vi "Autonomous Independent 3-17-15.vi"() -> ()   [LabVIEW 2014]
doc: "This VI is called when autonomous begins, and will automatically be terminated when autonomous ends. You can carry out timed or sensor driven robot movement independently without needing to return to the caller."
uses:
  Dashboard/Autonomous Type.ctl
  <vilib>/Rock Robotics/WPI/Joystick/WPI_JoystickGetSetRefNum.vi
  <vilib>/Rock Robotics/Network Tables/SD Write Numeric Array.vi
  <vilib>/Rock Robotics/WPI/RobotDrive/WPI_RobotDriveGetSetRefNum.vi
  <vilib>/Rock Robotics/Network Tables/SD Read Number.vi
  <vilib>/Rock Robotics/Network Tables/SD Write String.vi
  <vilib>/Rock Robotics/WPI/RobotDrive/WPI_RobotDriveMecanumDrive_Cartesian.vi
panel:
  in  "3 totes strafe":T1(array[cluster])=[{"X Joystick Value"=-0.3, "Y Joystick Value"=-1.0, "Z Joystick Value"=0.0, "Delay (sec)"=1.0, "Movement Name"="", "Mode"=enum."Move Robot"}, {"X Joystick Value"=0.3, "Y Joystick Value"=0.0, "Z Joystick Value"=0.0, "Delay (sec)"=0.25, "Movement Name"="", "Mode"=enum."Lift Tote"}, {"X Joystick Value"=0.0, "Y Joystick Value"=-0.5, "Z Joystick Value"=0.0, "Delay (sec)"=1.0, "Movement Name"="", "Mode"=enum."Move Robot"}, {"X Joystick Value"=0.0, "Y Joystick Value"=0.0, "Z Joystick Value"=0.0, "Delay (sec)"=4.0, "Movement Name"="", "Mode"=enum."Lift Tote"}, {"X Joystick Value"=0.0, "Y Joystick Value"=0.3, "Z Joystick Value"=0.0, "Delay (sec)"=1.0, "Movement Name"="", "Mode"=enum."Move Robot"}, {"X Joystick Value"=0.5353535353535355, "Y Joystick Value"=0.0, "Z Joystick Value"=0.0, "Delay (sec)"=1.0, "Movement Name"="", "Mode"=enum."Move Robot"}, {"X Joystick Value"=0.0, "Y Joystick Value"=-0.3, "Z Joystick Value"=0.0, "Delay (sec)"=0.251, "Movement Name"="", "Mode"=enum."Move Robot"}, {"X Joystick Value"=-0.3, "Y Joystick Value"=0.0, "Z Joystick Value"=0.0, "Delay (sec)"=1.0, "Movement Name"="", "Mode"=enum."Move Robot"}, {"X Joystick Value"=0.3, "Y Joystick Value"=0.0, "Z Joystick Value"=0.0, "Delay (sec)"=0.25, "Movement Name"="", "Mode"=enum."Move Robot"}, {"X Joystick Value"=0.0, "Y Joystick Value"=-0.5, "Z Joystick Value"=0.0, "Delay (sec)"=0.0, "Movement Name"="", "Mode"=enum."Move Robot"}, {"X Joystick Value"=0.0, "Y Joystick Value"=0.0, "Z Joystick Value"=0.0, "Delay (sec)"=3.5, "Movement Name"="", "Mode"=enum."Lift Tote"}, {"X Joystick Value"=0.0, "Y Joystick Value"=0.3, "Z Joystick Value"=0.0, "Delay (sec)"=3.5, "Movement Name"="", "Mode"=enum."Move Robot"}, {"X Joystick Value"=0.3, "Y Joystick Value"=0.0, "Z Joystick Value"=0.0, "Delay (sec)"=0.0, "Movement Name"="", "Mode"=enum."Move Robot"}, {"X Joystick Value"=0.0, "Y Joystick Value"=-0.5, "Z Joystick Value"=0.0, "Delay (sec)"=0.0, "Movement Name"="", "Mode"=enum."Move Robot"}, {"X Joystick Value"=-0.3, "Y Joystick Value"=0.0, "Z Joystick Value"=0.0, "Delay (sec)"=0.0, "Movement Name"="", "Mode"=enum."Move Robot"}, {"X Joystick Value"=0.3, "Y Joystick Value"=0.0, "Z Joystick Value"=0.0, "Delay (sec)"=0.0, "Movement Name"="", "Mode"=enum."Move Robot"}, {"X Joystick Value"=0.0, "Y Joystick Value"=-0.5, "Z Joystick Value"=0.0, "Delay (sec)"=0.0, "Movement Name"="", "Mode"=enum."Do Nothing"}, {"X Joystick Value"=0.0, "Y Joystick Value"=0.0, "Z Joystick Value"=0.0, "Delay (sec)"=0.0, "Movement Name"="", "Mode"=enum."Lift Tote"}, {"X Joystick Value"=0.0, "Y Joystick Value"=0.5, "Z Joystick Value"=0.0, "Delay (sec)"=0.0, "Movement Name"="", "Mode"=enum."Move Robot"}] {"Z Joystick Value" scale=-1.0..1.0; "Y Joystick Value" scale=1.0..-1.0; "X Joystick Value" scale=-1.0..1.0}
  in  "2 totes + turn":T1(array[cluster])=[{"X Joystick Value"=-0.3, "Y Joystick Value"=0.0, "Z Joystick Value"=0.0, "Delay (sec)"=1.0, "Movement Name"="", "Mode"=enum."Move Robot"}, {"X Joystick Value"=0.3, "Y Joystick Value"=0.0, "Z Joystick Value"=0.0, "Delay (sec)"=0.25, "Movement Name"="", "Mode"=enum."Move Robot"}, {"X Joystick Value"=0.0, "Y Joystick Value"=-0.5, "Z Joystick Value"=0.0, "Delay (sec)"=1.0, "Movement Name"="", "Mode"=enum."Move Robot"}, {"X Joystick Value"=0.0, "Y Joystick Value"=0.0, "Z Joystick Value"=0.0, "Delay (sec)"=4.0, "Movement Name"="", "Mode"=enum."Lift Tote"}, {"X Joystick Value"=0.0, "Y Joystick Value"=0.3, "Z Joystick Value"=0.0, "Delay (sec)"=0.30000000000000004, "Movement Name"="", "Mode"=enum."Move Robot"}, {"X Joystick Value"=0.0, "Y Joystick Value"=0.0, "Z Joystick Value"=0.677190686694989, "Delay (sec)"=2.0, "Movement Name"="", "Mode"=enum."Move Robot"}, {"X Joystick Value"=0.0, "Y Joystick Value"=-0.5, "Z Joystick Value"=0.0, "Delay (sec)"=2.0, "Movement Name"="", "Mode"=enum."Move Robot"}, {"X Joystick Value"=0.0, "Y Joystick Value"=0.0, "Z Joystick Value"=-0.6724763557187154, "Delay (sec)"=1.0, "Movement Name"="", "Mode"=enum."Move Robot"}, {"X Joystick Value"=0.0, "Y Joystick Value"=-0.5, "Z Joystick Value"=0.0, "Delay (sec)"=0.25, "Movement Name"="", "Mode"=enum."Move Robot"}, {"X Joystick Value"=-0.3, "Y Joystick Value"=0.0, "Z Joystick Value"=0.0, "Delay (sec)"=1.0, "Movement Name"="", "Mode"=enum."Move Robot"}, {"X Joystick Value"=0.3, "Y Joystick Value"=0.0, "Z Joystick Value"=0.0, "Delay (sec)"=0.0, "Movement Name"="", "Mode"=enum."Move Robot"}, {"X Joystick Value"=0.0, "Y Joystick Value"=-0.3, "Z Joystick Value"=0.0, "Delay (sec)"=0.0, "Movement Name"="", "Mode"=enum."Move Robot"}, {"X Joystick Value"=0.0, "Y Joystick Value"=0.0, "Z Joystick Value"=0.0, "Delay (sec)"=0.0, "Movement Name"="", "Mode"=enum."Lift Tote"}, {"X Joystick Value"=0.0, "Y Joystick Value"=0.3, "Z Joystick Value"=0.0, "Delay (sec)"=5.0, "Movement Name"="", "Mode"=enum."Move Robot"}, {"X Joystick Value"=0.0, "Y Joystick Value"=0.0, "Z Joystick Value"=0.67, "Delay (sec)"=0.0, "Movement Name"="", "Mode"=enum."Move Robot"}, {"X Joystick Value"=0.0, "Y Joystick Value"=-0.5, "Z Joystick Value"=0.0, "Delay (sec)"=0.0, "Movement Name"="", "Mode"=enum."Move Robot"}, {"X Joystick Value"=0.0, "Y Joystick Value"=0.0, "Z Joystick Value"=-0.67, "Delay (sec)"=0.0, "Movement Name"="", "Mode"=enum."Move Robot"}, {"X Joystick Value"=0.0, "Y Joystick Value"=-0.5, "Z Joystick Value"=0.0, "Delay (sec)"=0.0, "Movement Name"="", "Mode"=enum."Move Robot"}, {"X Joystick Value"=-0.3, "Y Joystick Value"=0.0, "Z Joystick Value"=0.0, "Delay (sec)"=0.0, "Movement Name"="", "Mode"=enum."Move Robot"}, {"X Joystick Value"=0.3, "Y Joystick Value"=0.0, "Z Joystick Value"=0.0, "Delay (sec)"=0.0, "Movement Name"="", "Mode"=enum."Move Robot"}, {"X Joystick Value"=0.0, "Y Joystick Value"=-0.5, "Z Joystick Value"=0.0, "Delay (sec)"=0.0, "Movement Name"="", "Mode"=enum."Move Robot"}, {"X Joystick Value"=0.0, "Y Joystick Value"=0.0, "Z Joystick Value"=0.0, "Delay (sec)"=0.0, "Movement Name"="", "Mode"=enum."Lift Tote"}, {"X Joystick Value"=0.0, "Y Joystick Value"=0.5, "Z Joystick Value"=0.0, "Delay (sec)"=0.0, "Movement Name"="", "Mode"=enum."Move Robot"}, {"X Joystick Value"=0.0, "Y Joystick Value"=-0.3, "Z Joystick Value"=0.0, "Delay (sec)"=0.0, "Movement Name"="", "Mode"=enum."Move Robot"}, {"X Joystick Value"=0.0, "Y Joystick Value"=0.0, "Z Joystick Value"=0.0, "Delay (sec)"=0.0, "Movement Name"="", "Mode"=enum."Lift Tote"}, {"X Joystick Value"=0.0, "Y Joystick Value"=0.5, "Z Joystick Value"=0.0, "Delay (sec)"=0.0, "Movement Name"="", "Mode"=enum."Move Robot"}] {"Z Joystick Value" scale=-1.0..1.0; "Y Joystick Value" scale=1.0..-1.0; "X Joystick Value" scale=-1.0..1.0}
  in  "do nothing":T1(array[cluster])=[{"X Joystick Value"=0.0, "Y Joystick Value"=0.0, "Z Joystick Value"=0.0, "Delay (sec)"=1.5, "Movement Name"="", "Mode"=enum."Do Nothing"}, {"X Joystick Value"=0.0, "Y Joystick Value"=0.0, "Z Joystick Value"=0.0, "Delay (sec)"=5.0, "Movement Name"="", "Mode"=enum."Move Robot"}, {"X Joystick Value"=0.0, "Y Joystick Value"=-1.0, "Z Joystick Value"=0.0, "Delay (sec)"=0.0, "Movement Name"="", "Mode"=enum."Move Robot"}, {"X Joystick Value"=-1.0, "Y Joystick Value"=0.0, "Z Joystick Value"=0.0, "Delay (sec)"=5.0, "Movement Name"="", "Mode"=enum."Totes Down"}, {"X Joystick Value"=0.0, "Y Joystick Value"=-1.0, "Z Joystick Value"=0.0, "Delay (sec)"=0.0, "Movement Name"="", "Mode"=enum."Do Nothing"}, {"X Joystick Value"=0.0, "Y Joystick Value"=0.0, "Z Joystick Value"=0.0, "Delay (sec)"=0.0, "Movement Name"="", "Mode"=enum."Do Nothing"}, {"X Joystick Value"=0.0, "Y Joystick Value"=-1.0, "Z Joystick Value"=0.0, "Delay (sec)"=0.0, "Movement Name"="", "Mode"=enum."Move Robot"}, {"X Joystick Value"=-1.0, "Y Joystick Value"=0.0, "Z Joystick Value"=0.0, "Delay (sec)"=0.0, "Movement Name"="", "Mode"=enum."Do Nothing"}, {"X Joystick Value"=0.0, "Y Joystick Value"=-1.0, "Z Joystick Value"=0.0, "Delay (sec)"=0.0, "Movement Name"="", "Mode"=enum."Do Nothing"}, {"X Joystick Value"=0.0, "Y Joystick Value"=0.0, "Z Joystick Value"=0.0, "Delay (sec)"=5.0, "Movement Name"="", "Mode"=enum."Do Nothing"}, {"X Joystick Value"=0.0, "Y Joystick Value"=-1.0, "Z Joystick Value"=0.0, "Delay (sec)"=0.0, "Movement Name"="", "Mode"=enum."Do Nothing"}, {"X Joystick Value"=0.0, "Y Joystick Value"=0.0, "Z Joystick Value"=0.0, "Delay (sec)"=0.0, "Movement Name"="", "Mode"=enum."Do Nothing"}] {"Z Joystick Value" scale=-1.0..1.0; "Y Joystick Value" scale=1.0..-1.0; "X Joystick Value" scale=-1.0..1.0}
  in  "3 totes + turn":T1(array[cluster])=[{"X Joystick Value"=-0.3, "Y Joystick Value"=0.0, "Z Joystick Value"=0.0, "Delay (sec)"=1.0, "Movement Name"="", "Mode"=enum."Move Robot"}, {"X Joystick Value"=0.3, "Y Joystick Value"=0.0, "Z Joystick Value"=0.0, "Delay (sec)"=0.25, "Movement Name"="", "Mode"=enum."Move Robot"}, {"X Joystick Value"=0.0, "Y Joystick Value"=-0.5, "Z Joystick Value"=0.0, "Delay (sec)"=1.0, "Movement Name"="", "Mode"=enum."Move Robot"}, {"X Joystick Value"=0.0, "Y Joystick Value"=0.0, "Z Joystick Value"=0.0, "Delay (sec)"=4.0, "Movement Name"="", "Mode"=enum."Lift Tote"}, {"X Joystick Value"=0.0, "Y Joystick Value"=0.3, "Z Joystick Value"=0.0, "Delay (sec)"=0.75, "Movement Name"="", "Mode"=enum."Move Robot"}, {"X Joystick Value"=0.0, "Y Joystick Value"=0.0, "Z Joystick Value"=0.677190686694989, "Delay (sec)"=1.5, "Movement Name"="", "Mode"=enum."Move Robot"}, {"X Joystick Value"=0.0, "Y Joystick Value"=-0.5, "Z Joystick Value"=0.0, "Delay (sec)"=1.5, "Movement Name"="", "Mode"=enum."Move Robot"}, {"X Joystick Value"=0.0, "Y Joystick Value"=0.0, "Z Joystick Value"=-0.6724763557187154, "Delay (sec)"=1.5, "Movement Name"="", "Mode"=enum."Move Robot"}, {"X Joystick Value"=0.0, "Y Joystick Value"=-0.5, "Z Joystick Value"=0.0, "Delay (sec)"=0.5, "Movement Name"="", "Mode"=enum."Move Robot"}, {"X Joystick Value"=-0.3, "Y Joystick Value"=0.0, "Z Joystick Value"=0.0, "Delay (sec)"=1.0, "Movement Name"="", "Mode"=enum."Move Robot"}, {"X Joystick Value"=0.3, "Y Joystick Value"=0.0, "Z Joystick Value"=0.0, "Delay (sec)"=0.25, "Movement Name"="", "Mode"=enum."Move Robot"}, {"X Joystick Value"=0.0, "Y Joystick Value"=-0.3, "Z Joystick Value"=0.0, "Delay (sec)"=1.0, "Movement Name"="", "Mode"=enum."Move Robot"}, {"X Joystick Value"=0.0, "Y Joystick Value"=0.0, "Z Joystick Value"=0.0, "Delay (sec)"=4.0, "Movement Name"="", "Mode"=enum."Lift Tote"}, {"X Joystick Value"=0.0, "Y Joystick Value"=0.3, "Z Joystick Value"=0.0, "Delay (sec)"=0.75, "Movement Name"="", "Mode"=enum."Move Robot"}, {"X Joystick Value"=0.0, "Y Joystick Value"=0.0, "Z Joystick Value"=0.67, "Delay (sec)"=1.5, "Movement Name"="", "Mode"=enum."Move Robot"}, {"X Joystick Value"=0.0, "Y Joystick Value"=-0.5, "Z Joystick Value"=0.0, "Delay (sec)"=1.5, "Movement Name"="", "Mode"=enum."Move Robot"}, {"X Joystick Value"=0.0, "Y Joystick Value"=0.0, "Z Joystick Value"=-0.67, "Delay (sec)"=1.5, "Movement Name"="", "Mode"=enum."Move Robot"}, {"X Joystick Value"=0.0, "Y Joystick Value"=-0.5, "Z Joystick Value"=0.0, "Delay (sec)"=0.5, "Movement Name"="", "Mode"=enum."Move Robot"}, {"X Joystick Value"=-0.3, "Y Joystick Value"=0.0, "Z Joystick Value"=0.0, "Delay (sec)"=1.0, "Movement Name"="", "Mode"=enum."Move Robot"}, {"X Joystick Value"=0.3, "Y Joystick Value"=0.0, "Z Joystick Value"=0.0, "Delay (sec)"=0.25, "Movement Name"="", "Mode"=enum."Move Robot"}, {"X Joystick Value"=0.0, "Y Joystick Value"=-0.5, "Z Joystick Value"=0.0, "Delay (sec)"=1.0, "Movement Name"="", "Mode"=enum."Move Robot"}, {"X Joystick Value"=0.0, "Y Joystick Value"=0.0, "Z Joystick Value"=0.0, "Delay (sec)"=4.0, "Movement Name"="", "Mode"=enum."Lift Tote"}, {"X Joystick Value"=0.0, "Y Joystick Value"=0.5, "Z Joystick Value"=0.0, "Delay (sec)"=4.0, "Movement Name"="", "Mode"=enum."Move Robot"}, {"X Joystick Value"=0.0, "Y Joystick Value"=-0.3, "Z Joystick Value"=0.0, "Delay (sec)"=0.0, "Movement Name"="", "Mode"=enum."Move Robot"}, {"X Joystick Value"=0.0, "Y Joystick Value"=0.0, "Z Joystick Value"=0.0, "Delay (sec)"=0.0, "Movement Name"="", "Mode"=enum."Lift Tote"}, {"X Joystick Value"=0.0, "Y Joystick Value"=0.5, "Z Joystick Value"=0.0, "Delay (sec)"=0.0, "Movement Name"="", "Mode"=enum."Move Robot"}] {"Z Joystick Value" scale=-1.0..1.0; "Y Joystick Value" scale=1.0..-1.0; "X Joystick Value" scale=-1.0..1.0}
  in  "move forward":T1(array[cluster])=[{"X Joystick Value"=0.0, "Y Joystick Value"=-0.3, "Z Joystick Value"=0.0, "Delay (sec)"=1.5, "Movement Name"="", "Mode"=enum."Move Robot"}, {"X Joystick Value"=0.0, "Y Joystick Value"=0.0, "Z Joystick Value"=0.0, "Delay (sec)"=5.0, "Movement Name"="", "Mode"=enum."Move Robot"}, {"X Joystick Value"=0.0, "Y Joystick Value"=-1.0, "Z Joystick Value"=0.0, "Delay (sec)"=0.0, "Movement Name"="", "Mode"=enum."Move Robot"}, {"X Joystick Value"=-1.0, "Y Joystick Value"=0.0, "Z Joystick Value"=0.0, "Delay (sec)"=5.0, "Movement Name"="", "Mode"=enum."Totes Down"}, {"X Joystick Value"=0.0, "Y Joystick Value"=-1.0, "Z Joystick Value"=0.0, "Delay (sec)"=0.0, "Movement Name"="", "Mode"=enum."Do Nothing"}, {"X Joystick Value"=0.0, "Y Joystick Value"=0.0, "Z Joystick Value"=0.0, "Delay (sec)"=0.0, "Movement Name"="", "Mode"=enum."Do Nothing"}, {"X Joystick Value"=0.0, "Y Joystick Value"=-1.0, "Z Joystick Value"=0.0, "Delay (sec)"=0.0, "Movement Name"="", "Mode"=enum."Move Robot"}, {"X Joystick Value"=-1.0, "Y Joystick Value"=0.0, "Z Joystick Value"=0.0, "Delay (sec)"=0.0, "Movement Name"="", "Mode"=enum."Do Nothing"}, {"X Joystick Value"=0.0, "Y Joystick Value"=-1.0, "Z Joystick Value"=0.0, "Delay (sec)"=0.0, "Movement Name"="", "Mode"=enum."Do Nothing"}, {"X Joystick Value"=0.0, "Y Joystick Value"=0.0, "Z Joystick Value"=0.0, "Delay (sec)"=5.0, "Movement Name"="", "Mode"=enum."Do Nothing"}, {"X Joystick Value"=0.0, "Y Joystick Value"=-1.0, "Z Joystick Value"=0.0, "Delay (sec)"=0.0, "Movement Name"="", "Mode"=enum."Do Nothing"}, {"X Joystick Value"=0.0, "Y Joystick Value"=0.0, "Z Joystick Value"=0.0, "Delay (sec)"=0.0, "Movement Name"="", "Mode"=enum."Do Nothing"}] {"Z Joystick Value" scale=-1.0..1.0; "Y Joystick Value" scale=1.0..-1.0; "X Joystick Value" scale=-1.0..1.0}
  in  "1 tote":T1(array[cluster])=[{"X Joystick Value"=-0.3, "Y Joystick Value"=0.0, "Z Joystick Value"=0.0, "Delay (sec)"=1.0, "Movement Name"="", "Mode"=enum."Move Robot"}, {"X Joystick Value"=0.3, "Y Joystick Value"=0.0, "Z Joystick Value"=0.0, "Delay (sec)"=0.25, "Movement Name"="", "Mode"=enum."Move Robot"}, {"X Joystick Value"=0.0, "Y Joystick Value"=-0.5, "Z Joystick Value"=0.0, "Delay (sec)"=1.0, "Movement Name"="", "Mode"=enum."Move Robot"}, {"X Joystick Value"=0.0, "Y Joystick Value"=0.0, "Z Joystick Value"=0.0, "Delay (sec)"=4.0, "Movement Name"="", "Mode"=enum."Lift Tote"}, {"X Joystick Value"=0.0, "Y Joystick Value"=0.3, "Z Joystick Value"=0.0, "Delay (sec)"=3.5, "Movement Name"="", "Mode"=enum."Move Robot"}, {"X Joystick Value"=0.0, "Y Joystick Value"=0.0, "Z Joystick Value"=0.0, "Delay (sec)"=3.5, "Movement Name"="", "Mode"=enum."Totes Down"}, {"X Joystick Value"=0.0, "Y Joystick Value"=0.5, "Z Joystick Value"=0.0, "Delay (sec)"=0.5, "Movement Name"="", "Mode"=enum."Move Robot"}, {"X Joystick Value"=-1.0, "Y Joystick Value"=0.0, "Z Joystick Value"=0.0, "Delay (sec)"=0.0, "Movement Name"="", "Mode"=enum."Do Nothing"}, {"X Joystick Value"=0.0, "Y Joystick Value"=-1.0, "Z Joystick Value"=0.0, "Delay (sec)"=0.0, "Movement Name"="", "Mode"=enum."Do Nothing"}, {"X Joystick Value"=0.0, "Y Joystick Value"=0.0, "Z Joystick Value"=0.0, "Delay (sec)"=5.0, "Movement Name"="", "Mode"=enum."Do Nothing"}, {"X Joystick Value"=0.0, "Y Joystick Value"=-1.0, "Z Joystick Value"=0.0, "Delay (sec)"=0.0, "Movement Name"="", "Mode"=enum."Do Nothing"}, {"X Joystick Value"=0.0, "Y Joystick Value"=0.0, "Z Joystick Value"=0.0, "Delay (sec)"=0.0, "Movement Name"="", "Mode"=enum."Do Nothing"}] {"Z Joystick Value" scale=-1.0..1.0; "Y Joystick Value" scale=1.0..-1.0; "X Joystick Value" scale=-1.0..1.0}
  in  "2 totes strafe":T1(array[cluster])=[{"X Joystick Value"=-0.3, "Y Joystick Value"=-1.0, "Z Joystick Value"=0.0, "Delay (sec)"=1.0, "Movement Name"="", "Mode"=enum."Move Robot"}, {"X Joystick Value"=0.3, "Y Joystick Value"=0.0, "Z Joystick Value"=0.0, "Delay (sec)"=0.25, "Movement Name"="", "Mode"=enum."Lift Tote"}, {"X Joystick Value"=0.0, "Y Joystick Value"=-0.5, "Z Joystick Value"=0.0, "Delay (sec)"=1.0, "Movement Name"="", "Mode"=enum."Move Robot"}, {"X Joystick Value"=0.0, "Y Joystick Value"=0.0, "Z Joystick Value"=0.0, "Delay (sec)"=0.0, "Movement Name"="", "Mode"=enum."Lift Tote"}, {"X Joystick Value"=0.0, "Y Joystick Value"=0.3, "Z Joystick Value"=0.0, "Delay (sec)"=1.0, "Movement Name"="", "Mode"=enum."Move Robot"}, {"X Joystick Value"=0.5353535353535355, "Y Joystick Value"=0.0, "Z Joystick Value"=0.0, "Delay (sec)"=1.0, "Movement Name"="", "Mode"=enum."Move Robot"}, {"X Joystick Value"=0.0, "Y Joystick Value"=-0.3, "Z Joystick Value"=0.0, "Delay (sec)"=0.251, "Movement Name"="", "Mode"=enum."Move Robot"}, {"X Joystick Value"=-0.3, "Y Joystick Value"=0.0, "Z Joystick Value"=0.0, "Delay (sec)"=1.0, "Movement Name"="", "Mode"=enum."Move Robot"}, {"X Joystick Value"=0.3, "Y Joystick Value"=-0.5, "Z Joystick Value"=0.0, "Delay (sec)"=0.25, "Movement Name"="", "Mode"=enum."Move Robot"}, {"X Joystick Value"=0.0, "Y Joystick Value"=-0.5, "Z Joystick Value"=0.0, "Delay (sec)"=0.0, "Movement Name"="", "Mode"=enum."Move Robot"}, {"X Joystick Value"=0.0, "Y Joystick Value"=0.0, "Z Joystick Value"=0.0, "Delay (sec)"=3.5, "Movement Name"="", "Mode"=enum."Lift Tote"}, {"X Joystick Value"=0.0, "Y Joystick Value"=0.3, "Z Joystick Value"=0.0, "Delay (sec)"=3.5, "Movement Name"="", "Mode"=enum."Move Robot"}] {"Z Joystick Value" scale=-1.0..1.0; "Y Joystick Value" scale=1.0..-1.0; "X Joystick Value" scale=-1.0..1.0}
  # "...."
  # "lift tote"
  # "move forward"
  # "turn right"
  # "strafe right"
  # "move backward"
  # "lift tote"
  # "turn left"
  # "strafe right"
  # "move forward"
  # "move backward"
  # "move backward"
  # "strafe left"
  # "move forward"
  # "lift tote"
  # "turn right"
  # "move forward"
  # "move forward"
  # "strafe left"
  # "turn left"
  # "strafe left"
  # "move forward"
  # "strafe right"
  # "move forward"
  # "move forward"
  # "lift tote"
  # "strafe left"
  # "strafe left"
  # "move backward"
  # "lift tote"
  # "move backward"
  # "strafe left"
  # "strafe right"
  # "strafe right"
  # "move forward"
  # "strafe right"
  # "move forward"
  # "strafe right"
  # "move forward"
  # "lift tote"
  # "move backward"
  # "move forward"
  # "strafe right"
  # "strafe left"
  # "move backward"
  # "turn right"
  # "move forward"
  # "strafe right"
  # "move forward"
  # "strafe right"
  # "move forward"
  # "lift tote"
  # "lift tote"
  # "move backward"
  # "strafe left"
  # "turn left"
  # "move forward"
  # "MAKE SURE TO MAKE YOUR CHANGES INTO DEFAULTS BEFORE CLOSING THE PROGRAM!!!!!!!!!!!!!"
  # "to do so, right click on the edge of \"Array of robot movements\" array control and then select Data Operations>Make Current Value Default"
  # "I'll say it again in a different way..."
  # "Be sure to right-click and choose Data Operations>>Make Current Value default if you want to save the array values with the VI"
  # "lift tote"
  # "move forward"
  # "strafe right"
  # "move forward"
  # "move forward"
  # "lift tote"
  # "move backward"
  # "strafe right"
  # "move backward"
  # "strafe left"
  # "strafe left"
  # "strafe right"
  # "strafe left"
  # "strafe right"
  # "move forward"
  # "move backward"
  # "lift tote"
  # "move forward"
  # "do nothing"
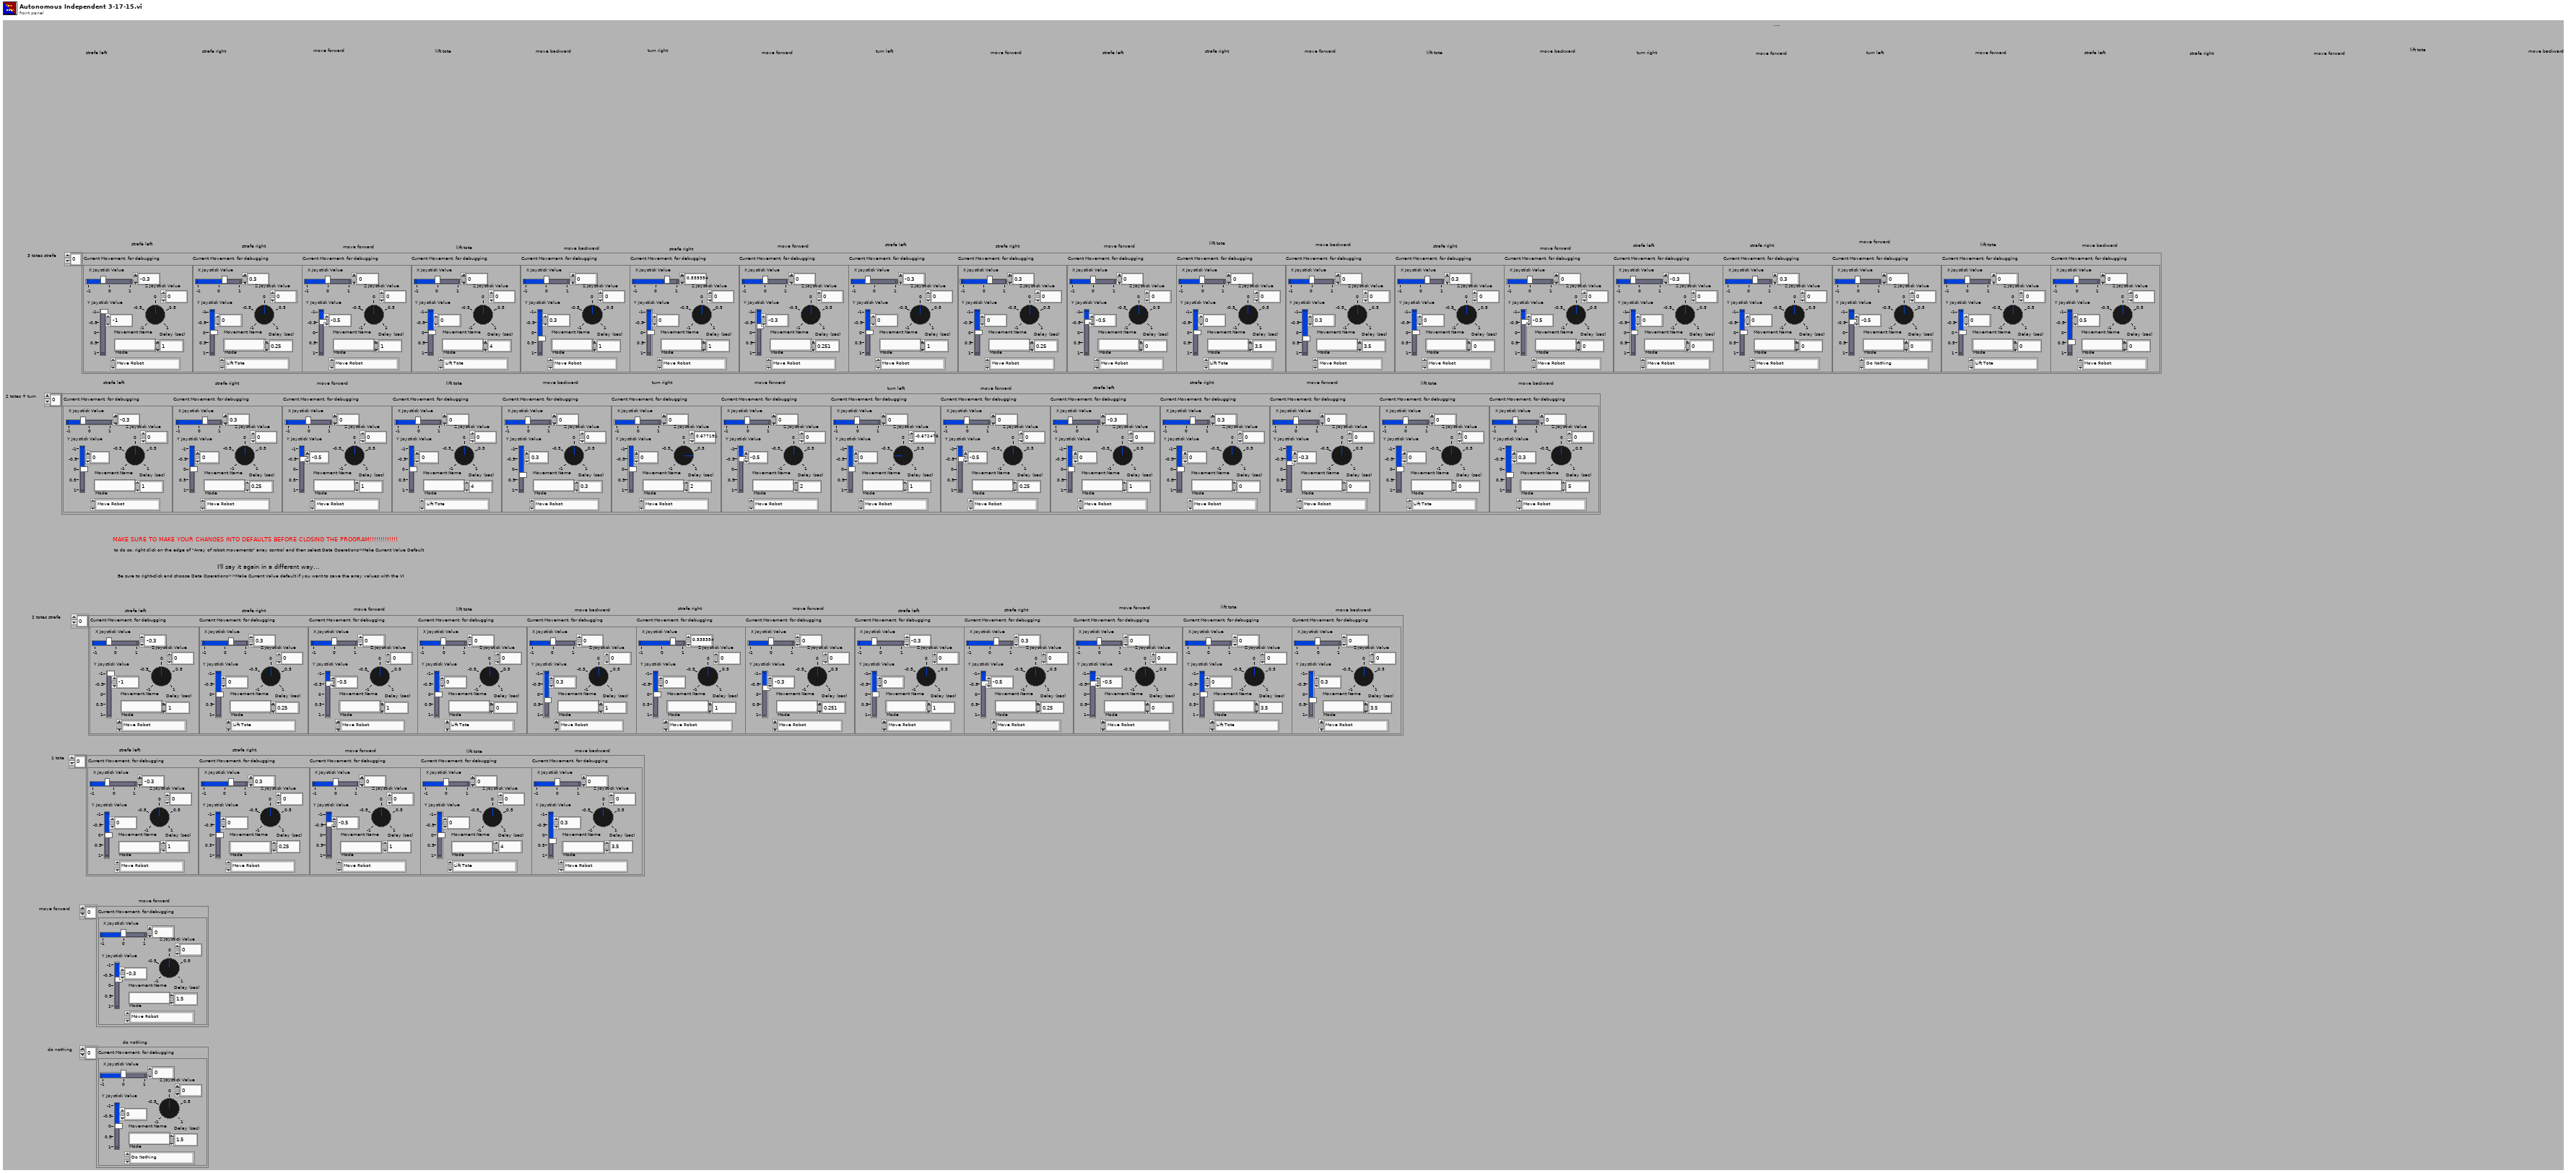
[diagram p1: front panel]
types:
  T1 = cluster{"X Joystick Value":dbl, "Y Joystick Value":dbl, "Z Joystick Value":dbl, "Delay (sec)":dbl, "Movement Name":string, "Mode":enum16{"Do Nothing", "Move Robot", "Lift Tote", "Totes Down", "Totes Up"}}[]
  T2 = typedef "Autonomous Type.ctl" = enum16{"2 Totes + Turn", "Nothing", "3 Totes + Turn", "3 Totes", "2 Totes", "1 Tote", "Forward"}
  T3 = typedef "WPI_JoystickDevRef.ctl" = cluster{"Device":T4}
  T4 = typedef "WPI_JoystickDeviceEnum.ctl" = enum16{"USB 0", "USB 1", "USB 2", "USB 3", "USB 4", "USB 5"}
  T5 = typedef "WPI_RobotDriveDevRef.ctl" = cluster{"DevStatus":errorcluster, "Motors[]":T6[], "Square Inputs":bool, "Max Output":dbl}
  T6 = typedef "WPI_MotorControlDeviceRef.ctl" = cluster{"DeviceStatus":errorcluster, "Type":T7, "PWM":cluster{"Controller":T8, "PWM Channel":T9, "DeadBand":T10}, "CAN":cluster{"Device Number":u8, "Control Mode":T11, "Semaphore":T12, "Max Vout":dbl, "TalonSRX Control Mode":T13}, "Invert":bool, "TransformRef":T14, "InvTransformRef":T14}
  T7 = typedef "WPI_MotorControlType.ctl" = enum16{"PWM", "CAN", "CANTalonSRX"}
  T8 = typedef "FPGA_TypedefDigitalModule.ctl" = enum16{"Controller 1"}
  T9 = typedef "FPGA_DIOPWMChannel.ctl" = enum8{"PWM 0", "PWM 1", "PWM 2", "PWM 3", "PWM 4", "PWM 5", "PWM 6", "PWM 7", "PWM 8", "PWM 9", "PWM MXP 0", "PWM MXP 1", "PWM MXP 2", "PWM MXP 3", "PWM MXP 4", "PWM MXP 5", "PWM MXP 6", "PWM MXP 7", "PWM MXP 8", "PWM MXP 9", "Invalid"}
  T10 = typedef "WPI_PWMDeadband.ctl" = cluster{"Name":string, "maxPositivePwm":i32, "minPositivePwm":i32, "centerPwm":i32, "maxNegativePwm":i32, "minNegativePwm":i32, "angularRange":u16}
  T11 = typedef "WPI_CANJaguar_ControlMode.ctl" = enum8{"Percent VBus", "Current", "Speed", "Position", "Voltage"}
  T12 = typedef "Semaphore RefNum" = refnum<k1>
  T13 = typedef "WPI_CANTalonSRX_APIControlMode.ctl" = enum8{"Percent VBus", "Speed", "Position", "Slave", "Unchanged / Invalid"}
  T14 = typedef "WPI_PWMTransform_ConPane.ctl" = refnum<vi>
  T15 = enum16{"Do Nothing", "Move Robot", "Lift Tote", "Totes Down", "Totes Up"}
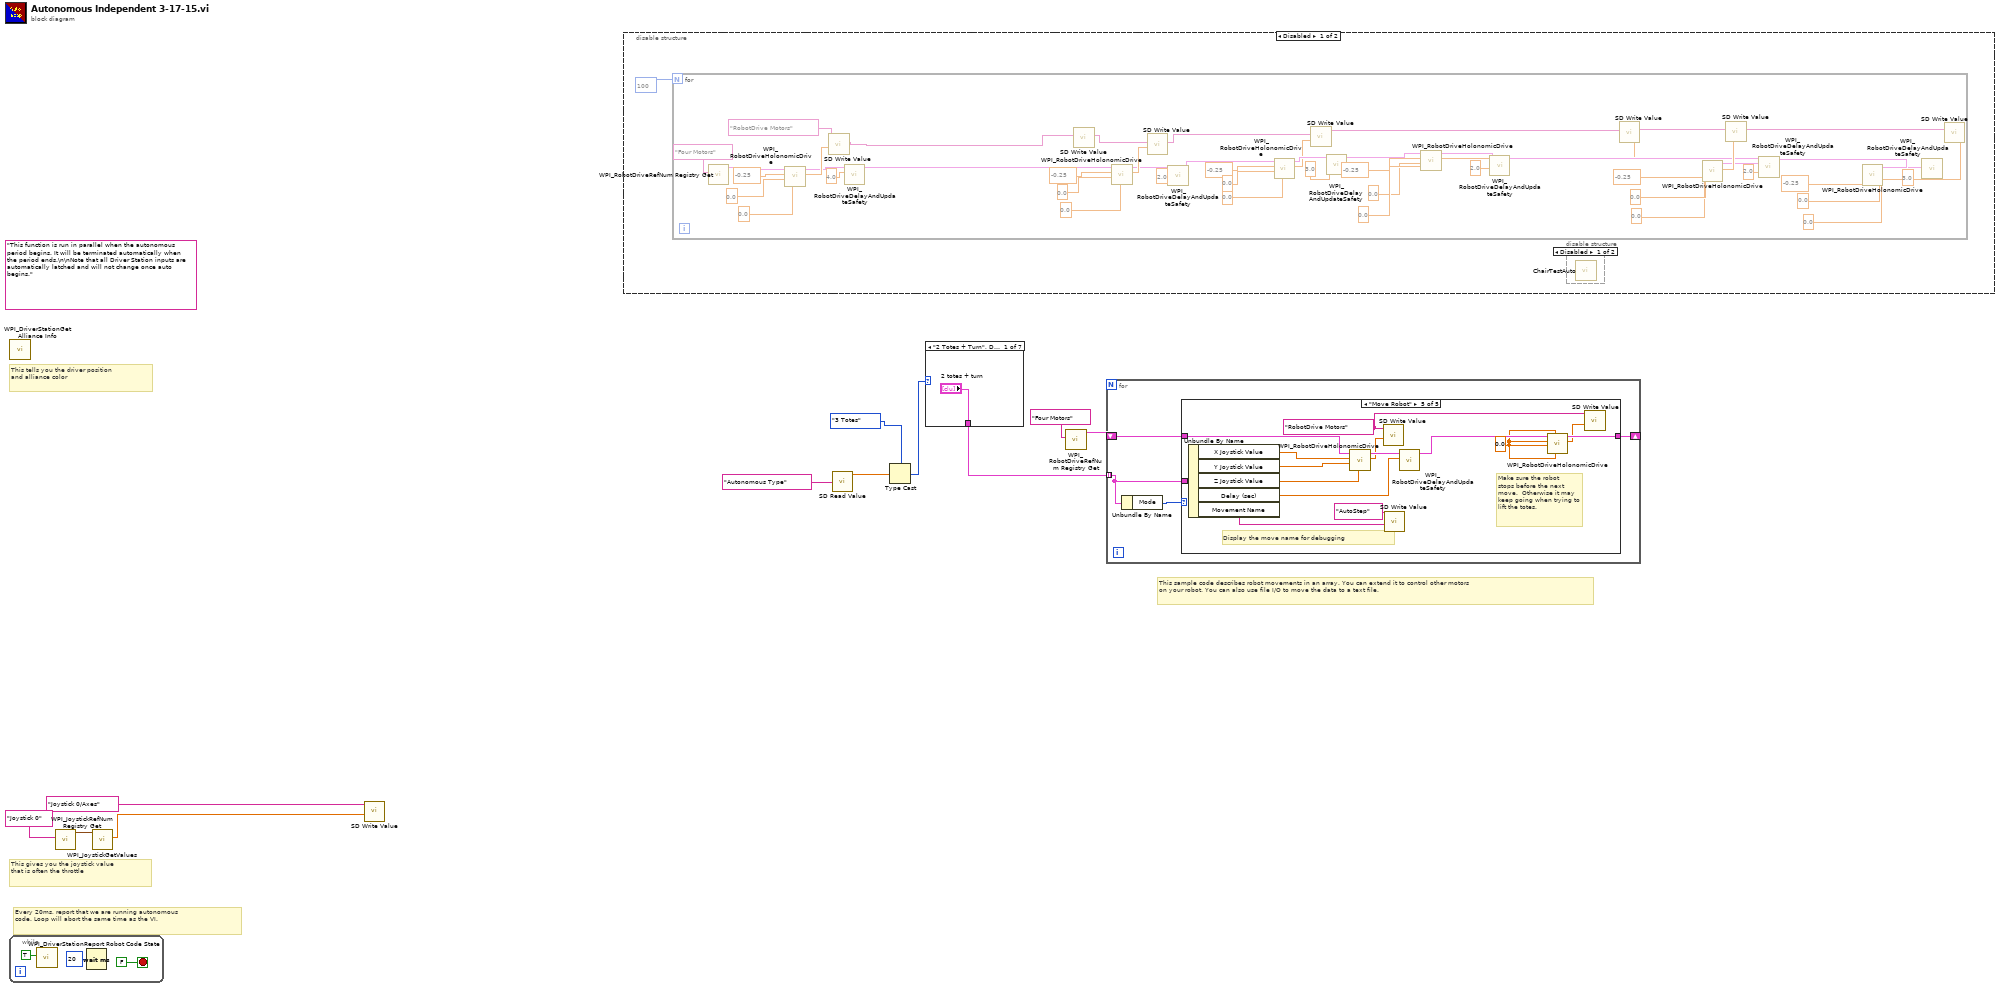
[diagram p0: block diagram]
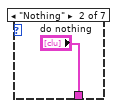
[diagram p2: hidden frame]
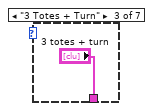
[diagram p3: hidden frame]
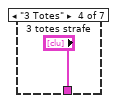
[diagram p4: hidden frame]
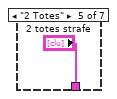
[diagram p5: hidden frame]
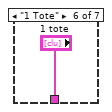
[diagram p6: hidden frame]
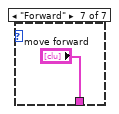
[diagram p7: hidden frame]
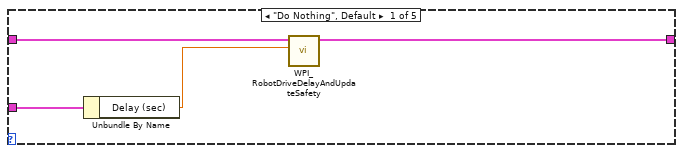
[diagram p8: hidden frame]
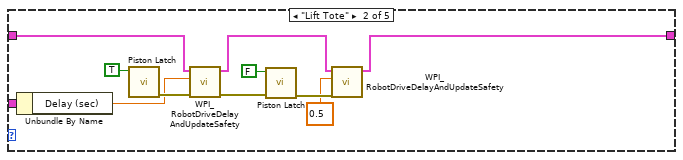
[diagram p9: hidden frame]
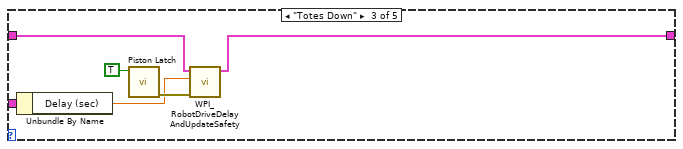
[diagram p10: hidden frame]
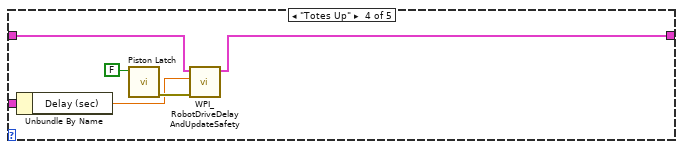
[diagram p11: hidden frame]
diagram:
  (unwired) "This function is run in parallel when the autonomous period begins. It will be terminated automatically when the period ends.\n\nNote that all Driver Station inputs are automatically latched and will not change once auto begins."
  # "This sample code describes robot movements in an array. You can extend it to control other motors\non your robot. You can also use file I/O to move the data to a text file."
  # "Every 20ms, report that we are running autonomous\ncode. Loop will abort the same time as the VI."
  # "This gives you the joystick value\nthat is often the throttle"
  # "This tells you the driver position\nand alliance color"
  n1 = while {
    stop <- FALSE stop-if-true
    n2 = call <vilib>:"WPI_DriverStationReport Robot Code State.vi"("Autonomous"=TRUE) -> ()  [unwired: 10 in, 1 out]
    n3 = Wait (ms)(milliseconds to wait=u32 20) -> ()  [unwired: 1 out]
  }
  n4 = call <vilib>:"WPI_DriverStationGet Alliance Info.vi"() -> ()  [unwired: 12 out]
  n5 = call <vilib>:"WPI_JoystickRefNum Registry Get.vi"("refnum name"="Joystick 0") -> ("JoystickDevRef"=w10:T3)  [unwired: 1 in, 9 out]
  n6 = call <vilib>:"WPI_JoystickGetValues.vi"("JoystickDevRef"=w10) -> ("Axes"=w8:dbl[])  [unwired: 6 in, 4 out]
  n7 = call-poly <vilib>:"SD Write Value.vi"("Numeric Array"=w8, "Name"="Joystick 0/Axes") -> ()  [unwired: 8 in, 2 out]
  n8 = disable-structure shown="Disabled" {
    frame Disabled {
      n9 = for {
        N: 100 -> [_]
        n10 = call <vilib>:"WPI_RobotDriveRefNum Registry Get.vi"("refnum name"="Four Motors") -> ("RobotDriveDevRef"=w34:T5)  [unwired: 1 in, 9 out]
        n11 = call-poly <vilib>:"WPI_RobotDriveHolonomicDrive.vi"("Rotation"=0.0, "Y"=0.0 ("X axis value"), "X"=-0.25 ("X axis value"), "RobotDriveDevRef"=w34) -> ("Motor Values"=w38:dbl[], "RobotDriveDevRef"=w28:T5)  [unwired: 5 in, 1 out]
        n12 = call-poly <vilib>:"SD Write Value.vi"("Numeric Array"=w38, "Name"="RobotDrive Motors") -> ("Table Prefix out"=w16:string)  [unwired: 8 in, 1 out]
        n13 = call <vilib>:"WPI_RobotDriveDelayAndUpdateSafety.vi"("Delay (s)"=4.0, "RobotDriveDevRef"=w28) -> ("RobotDriveDevRef 2"=w17:T5)  [unwired: 8 in, 1 out]
        n14 = call-poly <vilib>:"SD Write Value.vi"("Table Prefix"=w16) -> ("Table Prefix out"=w19:string)  [unwired: 9 in, 1 out]
        n15 = call-poly <vilib>:"WPI_RobotDriveHolonomicDrive.vi"("Rotation"=0.0, "Y"=0.0 ("X axis value"), "X"=-0.25 ("X axis value"), "RobotDriveDevRef"=w17) -> ("Motor Values"=w39:dbl[], "RobotDriveDevRef"=w29:T5)  [unwired: 5 in, 1 out]
        n16 = call-poly <vilib>:"SD Write Value.vi"("Numeric Array"=w39, "Table Prefix"=w19) -> ("Table Prefix out"=w18:string)  [unwired: 8 in, 1 out]
        n17 = call <vilib>:"WPI_RobotDriveDelayAndUpdateSafety.vi"("Delay (s)"=2.0, "RobotDriveDevRef"=w29) -> ("RobotDriveDevRef 2"=w30:T5)  [unwired: 8 in, 1 out]
        n18 = call-poly <vilib>:"WPI_RobotDriveHolonomicDrive.vi"("Rotation"=0.0 ("X axis value"), "Y"=0.0 ("X axis value"), "X"=-0.25 ("X axis value"), "RobotDriveDevRef"=w30) -> ("Motor Values"=w40:dbl[], "RobotDriveDevRef"=w42:T5)  [unwired: 5 in, 1 out]
        n19 = call-poly <vilib>:"SD Write Value.vi"("Numeric Array"=w40, "Table Prefix"=w18) -> ("Table Prefix out"=w49:string)  [unwired: 8 in, 1 out]
        n20 = call <vilib>:"WPI_RobotDriveDelayAndUpdateSafety.vi"("Delay (s)"=3.0, "RobotDriveDevRef"=w42) -> ("RobotDriveDevRef 2"=w43:T5)  [unwired: 8 in, 1 out]
        n21 = call-poly <vilib>:"WPI_RobotDriveHolonomicDrive.vi"("Rotation"=0.0, "Y"=0.0, "X"=-0.25, "RobotDriveDevRef"=w43) -> ("Motor Values"=w50:dbl[], "RobotDriveDevRef"=w47:T5)  [unwired: 5 in, 1 out]
        n22 = call <vilib>:"WPI_RobotDriveDelayAndUpdateSafety.vi"("Delay (s)"=2.0, "RobotDriveDevRef"=w47) -> ("RobotDriveDevRef 2"=w51:T5)  [unwired: 8 in, 1 out]
        n23 = call-poly <vilib>:"SD Write Value.vi"("Numeric Array"=w50, "Table Prefix"=w49) -> ("Table Prefix out"=w61:string)  [unwired: 8 in, 1 out]
        n24 = call-poly <vilib>:"WPI_RobotDriveHolonomicDrive.vi"("Rotation"=0.0, "Y"=0.0, "X"=-0.25, "RobotDriveDevRef"=w51) -> ("Motor Values"=w63:dbl[], "RobotDriveDevRef"=w55:T5)  [unwired: 5 in, 1 out]
        n25 = call-poly <vilib>:"SD Write Value.vi"("Numeric Array"=w63, "Table Prefix"=w61) -> ("Table Prefix out"=w65:string)  [unwired: 8 in, 1 out]
        n26 = call <vilib>:"WPI_RobotDriveDelayAndUpdateSafety.vi"("Delay (s)"=2.0, "RobotDriveDevRef"=w55) -> ("RobotDriveDevRef 2"=w62:T5)  [unwired: 8 in, 1 out]
        n27 = call-poly <vilib>:"WPI_RobotDriveHolonomicDrive.vi"("Rotation"=0.0, "Y"=0.0, "X"=-0.25, "RobotDriveDevRef"=w62) -> ("Motor Values"=w64:dbl[], "RobotDriveDevRef"=w59:T5)  [unwired: 5 in, 1 out]
        n28 = call <vilib>:"WPI_RobotDriveDelayAndUpdateSafety.vi"("Delay (s)"=3.0, "RobotDriveDevRef"=w59) -> ()  [unwired: 8 in, 2 out]
        n29 = call-poly <vilib>:"SD Write Value.vi"("Numeric Array"=w64, "Table Prefix"=w65) -> ()  [unwired: 8 in, 2 out]
      }
      n30 = disable-structure shown="Disabled" {
        frame Disabled {
          n31 = call "ChairTestAuto.vi"() -> ()  [unwired: 12 in]
        }
        frame Enabled {
        }
      }
    }
    frame Enabled {
    }
  }
  n32 = call-poly <vilib>:"SD Read Value.vi"("Name"="Autonomous Type") -> ("Numeric"=w4:dbl)  [unwired: 8 in, 2 out]
  n33 = Type Cast(type=Autonomous_Type."3 Totes" ("Auto Type"), x=w4) -> (*(type *) &x=w2:T2)
  n34 = case shown="\"2 Totes + Turn\", Default" w2 {
    tunnel: ["2 totes + turn" "do nothing" "3 totes + turn" "3 totes strafe" "2 totes strafe" "1 tote" "move forward"] -> w1
    frame "2 Totes + Turn", Default {
    }
    frame "Nothing" {
    }
    frame "3 Totes + Turn" {
    }
    frame "3 Totes" {
    }
    frame "2 Totes" {
    }
    frame "1 Tote" {
    }
    frame "Forward" {
    }
  }
  n35 = call <vilib>:"WPI_RobotDriveRefNum Registry Get.vi"("refnum name"="Four Motors") -> ("RobotDriveDevRef"=w6:T5)  [unwired: 1 in, 9 out]
  n36 = for {
    shift-right: [w75] -> _
    shift-left: w6 -> [w76]
    tunnel: w1 -> [w74] mode=indexing
    n37 = Unbundle By Name(w74) -> ("Mode"=w73:T15)
    n38 = case shown="\"Move Robot\"" w73 {
      tunnel: w76 -> [w79 w89 w95 w101 w117]
      tunnel: [w80 w84 w92 w98 w107] -> w75
      tunnel: w74 -> [w78 w82 w94 w100 w113]
      frame "Do Nothing", Default {
        n39 = Unbundle By Name(w78) -> ("Delay (sec)"=w77:dbl)
        n40 = call <vilib>:"WPI_RobotDriveDelayAndUpdateSafety.vi"("Delay (s)"=w77, "RobotDriveDevRef"=w79) -> ("RobotDriveDevRef 2"=w80:T5)  [unwired: 8 in, 1 out]
      }
      frame "Lift Tote" {
        n41 = Unbundle By Name(w82) -> ("Delay (sec)"=w81:dbl)
        n42 = call "Piston Latch.vi"("button value"=TRUE) -> ("error out"=w90:errorcluster)  [unwired: 10 in]
        n43 = call <vilib>:"WPI_RobotDriveDelayAndUpdateSafety.vi"("error in (no error)"=w90, "Delay (s)"=w81, "RobotDriveDevRef"=w89) -> ("error out"=w87:errorcluster, "RobotDriveDevRef 2"=w85:T5)  [unwired: 7 in]
        n44 = call "Piston Latch.vi"("error in (no error)"=w87, "button value"=FALSE) -> ("error out"=w86:errorcluster)  [unwired: 9 in]
        n45 = call <vilib>:"WPI_RobotDriveDelayAndUpdateSafety.vi"("error in (no error)"=w86, "Delay (s)"=0.5, "RobotDriveDevRef"=w85) -> ("RobotDriveDevRef 2"=w84:T5)  [unwired: 7 in, 1 out]
      }
      frame "Totes Down" {
        n46 = Unbundle By Name(w94) -> ("Delay (sec)"=w93:dbl)
        n47 = call "Piston Latch.vi"("button value"=TRUE) -> ("error out"=w96:errorcluster)  [unwired: 10 in]
        n48 = call <vilib>:"WPI_RobotDriveDelayAndUpdateSafety.vi"("error in (no error)"=w96, "Delay (s)"=w93, "RobotDriveDevRef"=w95) -> ("RobotDriveDevRef 2"=w92:T5)  [unwired: 7 in, 1 out]
      }
      frame "Totes Up" {
        n49 = Unbundle By Name(w100) -> ("Delay (sec)"=w99:dbl)
        n50 = call "Piston Latch.vi"("button value"=FALSE) -> ("error out"=w102:errorcluster)  [unwired: 10 in]
        n51 = call <vilib>:"WPI_RobotDriveDelayAndUpdateSafety.vi"("error in (no error)"=w102, "Delay (s)"=w99, "RobotDriveDevRef"=w101) -> ("RobotDriveDevRef 2"=w98:T5)  [unwired: 7 in, 1 out]
      }
      frame "Move Robot" {
        w106 = 0.0 ("X")
        w105 = "RobotDrive Motors" ("Name")
        # "Display the move name for debugging"
        # "Make sure the robot stops before the next move.  Otherwise it may keep going when trying to lift the totes."
        n52 = Unbundle By Name(w113) -> ("X Joystick Value"=w116:dbl, "Y Joystick Value"=w115:dbl, "Z Joystick Value"=w112:dbl, "Delay (sec)"=w114:dbl, "Movement Name"=w110:string)
        n53 = call-poly <vilib>:"WPI_RobotDriveHolonomicDrive.vi"("Rotation"=w112, "Y"=w115, "X"=w116, "RobotDriveDevRef"=w117) -> ("Motor Values"=w111:dbl[], "RobotDriveDevRef"=w118:T5)  [unwired: 5 in, 1 out]
        n54 = call-poly <vilib>:"SD Write Value.vi"("Numeric Array"=w111, "Name"=w105) -> ()  [unwired: 8 in, 2 out]
        n55 = call-poly <vilib>:"SD Write Value.vi"("String"=w110, "Name"="AutoStep") -> ()  [unwired: 8 in, 2 out]
        n56 = call <vilib>:"WPI_RobotDriveDelayAndUpdateSafety.vi"("Delay (s)"=w114, "RobotDriveDevRef"=w118) -> ("RobotDriveDevRef 2"=w108:T5)  [unwired: 8 in, 1 out]
        n57 = call-poly <vilib>:"WPI_RobotDriveHolonomicDrive.vi"("Rotation"=w106, "Gyro Angle"=w106, "Y"=w106, "X"=w106, "RobotDriveDevRef"=w108) -> ("Motor Values"=w104:dbl[], "RobotDriveDevRef"=w107:T5)  [unwired: 4 in, 1 out]
        n58 = call-poly <vilib>:"SD Write Value.vi"("Numeric Array"=w104, "Name"=w105) -> ()  [unwired: 8 in, 2 out]
      }
    }
  }
